vi "E2 Data Logger.vi"(7 "refnum in":refnum<file>) -> (3 "refnum out":refnum<file>)   [LabVIEW 2015]
uses:
  <vilib>/Rock Robotics/WPI/DriverStation/WPI_DriverStationRobotMode2.ctl
  Team Code/Robot Global Data.vi
  Moose Code/Auto_Conf.vi
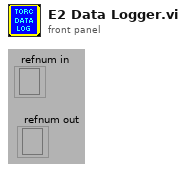
[diagram p1: front panel]
types:
  T1 = typedef "WPI_DriverStationRobotMode2.ctl" = enum16{"Autonomous Disabled", "Autonomous Enabled", "Teleop Disabled", "Teleop Enabled", "Disconnected", "Finish", "Test Disabled", "Test Enabled", "Emergency Stopped"}
  T2 = cluster{"LinearAcceleration X":dbl, "LinearAcceleration Y":dbl, "LinearAcceleration Z":dbl}
  T3 = cluster{"Velocity X":dbl, "Velocity Y":dbl, "Velocity Z":dbl, "Displacement X":dbl, "Displacement Y":dbl, "Displacement Z":dbl}
  T4 = enum16{"ResetBack", "ResetForward", "Reset", "Hold", "HighGoal", "LowGoal", "BumperShot", "EmergencyManualControl"}
  T5 = enum16{"ResetBack", "EmergencyManualControl", "ResetForward", "Hold", "Reset", "ManualControl"}
  T6 = cluster{"Yaw":dbl, "Roll":dbl, "Pitch":dbl, "Heading":dbl, "Fused Heading":dbl}
  T7 = typedef "WPI_SolenoidValue.ctl" = enum16{"Off", "On", "Forward", "Reverse"}
  T8 = typedef "WPI_CANTalonSRX_APIControlMode.ctl" = enum8{"Percent VBus", "Speed", "Position", "Slave", "Unchanged / Invalid", "Voltage Compensation", "Current", "Motion Profile"}
  T9 = enum16{"Empty", "Suck", "Hold", "LowGoal", "HighGoal", "BumperShot", "Shoot", "Dwell"}
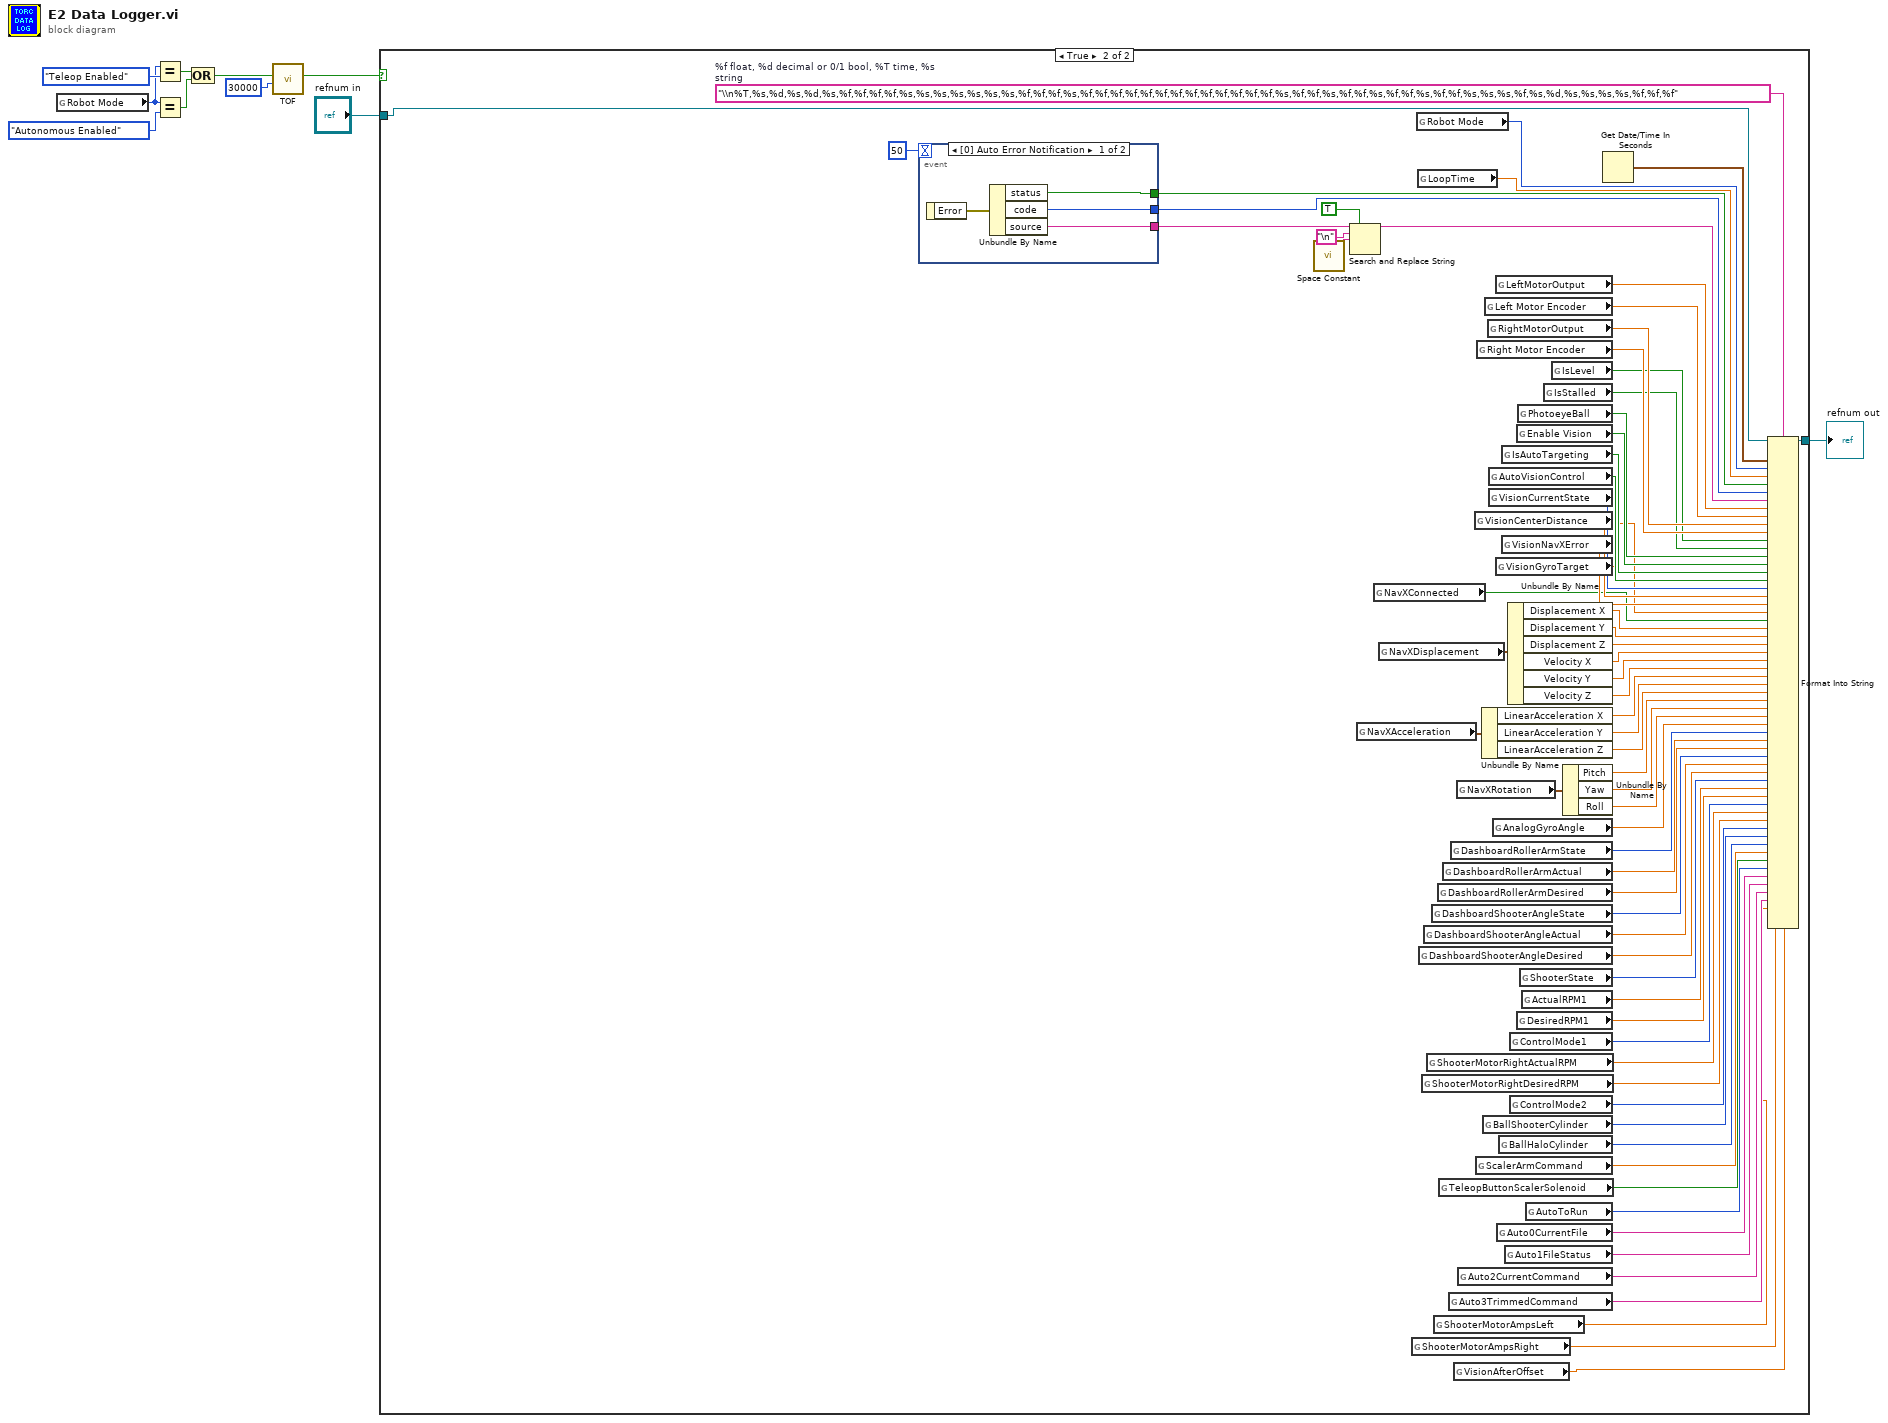
[diagram p0: block diagram]
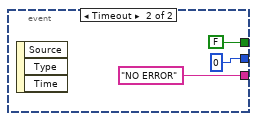
[diagram p3: hidden frame]
diagram:
  n1 = global read "Robot Global Data.vi" "Robot Mode"() -> (w4:T1)
  n2 = Equal?(x=w4, y=WPI_DriverStationRobotMode2."Teleop Enabled") -> (x = y?=w6:bool)
  n3 = Equal?(x=w4, y=WPI_DriverStationRobotMode2."Autonomous Enabled") -> (x = y?=w5:bool)
  n4 = Compound Arithmetic op=OR(w6, w5) -> (w3:bool)
  n5 = call "TOF.vi"("Delay (ms)"=u32 30000, "Input"=w3) -> ("Output"=w2:bool)  [unwired: 9 in]
  n6 = case shown="True" w2 {
    tunnel: [w11 w81] -> w10
    tunnel: "refnum in" -> [w11 w78]
    frame False {
    }
    frame True {
      w79 = "\\n%T,%s,%d,%s,%d,%s,%f,%f,%f,%f,%s,%s,%s,%s,%s,%s,%s,%f,%f,%f,%s,%f,%f,%f,%f,%f,%f,%f,%f,%f,%f,%f,%f,%f,%s,%f,%f,%s,%f,%f,%s,%f,%f,%s,%f,%f,%s,%s,%s,%f,%s,%d,%s,%s,%s,%s,%f,%f,%f"  # %f float, %d decimal or 0/1 bool, %T time, %s string
      n7 = event shown="[0] Auto Error Notification" {
        selector: _ -> [_ _]
        dyn-events: _ -> [_ _]
        timeout: 50 -> [_ _]
        tunnel: [w84 "NO ERROR" ("source")] -> w71
        tunnel: [w83 0 ("code")] -> w75
        tunnel: [w82 FALSE ("status")] -> w76
        event Auto Error Notification {
          n8 = event-data() -> ("Error"=w85:errorcluster)  [unwired: 1 in]
          n9 = Unbundle By Name(w85) -> ("status"=w82:bool, "code"=w83:i32, "source"=w84:string)
        }
        event Timeout {
          n10 = event-data() -> ()  [unwired: 1 in, 3 out]
        }
      }
      n11 = call <vilib>:"Space Constant.vi"() -> ("String"=w69:string)
      n12 = Search and Replace String(replace all?=TRUE ("replace all? (F)"), input string=w71, search string="\n", replace string=w69) -> (result string=w72:string)  [unwired: 4 in, 3 out]
      n13 = global read "Robot Global Data.vi" "NavXAcceleration"() -> (w73:T2)
      n14 = global read "Robot Global Data.vi" "NavXConnected"() -> (w52:bool)
      n15 = global read "Robot Global Data.vi" "NavXDisplacement"() -> (w51:T3)
      n16 = global read "Robot Global Data.vi" "ShooterMotorAmpsRight"() -> (w16:dbl)
      n17 = global read "Robot Global Data.vi" "Robot Mode"() -> (w18:T1)
      n18 = global read "Robot Global Data.vi" "LoopTime"() -> (w67:dbl)
      n19 = global read "Robot Global Data.vi" "DashboardShooterAngleDesired"() -> (w35:dbl)
      n20 = global read "Robot Global Data.vi" "ShooterMotorRightDesiredRPM"() -> (w29:dbl)
      n21 = global read "Robot Global Data.vi" "DashboardShooterAngleActual"() -> (w36:dbl)
      n22 = global read "Robot Global Data.vi" "ShooterMotorRightActualRPM"() -> (w30:dbl)
      n23 = global read "Robot Global Data.vi" "DashboardShooterAngleState"() -> (w37:T4)
      n24 = global read "Robot Global Data.vi" "ShooterMotorAmpsLeft"() -> (w17:dbl)
      n25 = global read "Robot Global Data.vi" "DashboardRollerArmDesired"() -> (w38:dbl)
      n26 = global read "Robot Global Data.vi" "TeleopButtonScalerSolenoid"() -> (w19:bool)
      n27 = global read "Robot Global Data.vi" "DashboardRollerArmActual"() -> (w39:dbl)
      n28 = global read "Auto_Conf.vi" "Auto3TrimmedCommand"() -> (w20:string)
      n29 = global read "Robot Global Data.vi" "DashboardRollerArmState"() -> (w40:T5)
      n30 = global read "Robot Global Data.vi" "VisionAfterOffset"() -> (w12:dbl)
      n31 = global read "Robot Global Data.vi" "NavXRotation"() -> (w74:T6)
      n32 = global read "Auto_Conf.vi" "Auto2CurrentCommand"() -> (w21:string)
      n33 = global read "Robot Global Data.vi" "VisionCenterDistance"() -> (w55:dbl)
      n34 = global read "Robot Global Data.vi" "ScalerArmCommand"() -> (w25:dbl)
      n35 = global read "Robot Global Data.vi" "Right Motor Encoder"() -> (w63:dbl)
      n36 = Unbundle By Name(w73) -> ("LinearAcceleration X"=w44:dbl, "LinearAcceleration Y"=w43:dbl, "LinearAcceleration Z"=w42:dbl)
      n37 = global read "Robot Global Data.vi" "BallShooterCylinder"() -> (w27:T7)
      n38 = global read "Robot Global Data.vi" "Left Motor Encoder"() -> (w65:dbl)
      n39 = global read "Robot Global Data.vi" "RightMotorOutput"() -> (w64:dbl)
      n40 = global read "Robot Global Data.vi" "AutoVisionControl"() -> (w57:bool)
      n41 = global read "Robot Global Data.vi" "VisionCurrentState"() -> (w56:enum16{"Disabled", "Enable", "Suspended", "PID"})
      n42 = global read "Robot Global Data.vi" "AnalogGyroAngle"() -> (w41:dbl)
      n43 = global read "Robot Global Data.vi" "LeftMotorOutput"() -> (w66:dbl)
      n44 = global read "Robot Global Data.vi" "VisionGyroTarget"() -> (w53:dbl)
      n45 = global read "Auto_Conf.vi" "Auto0CurrentFile"() -> (w23:string)
      n46 = global read "Robot Global Data.vi" "BallHaloCylinder"() -> (w26:T7)
      n47 = global read "Robot Global Data.vi" "IsAutoTargeting"() -> (w58:bool)
      n48 = global read "Robot Global Data.vi" "VisionNavXError"() -> (w54:dbl)
      n49 = global read "Auto_Conf.vi" "Auto1FileStatus"() -> (w22:string)
      n50 = Unbundle By Name(w51) -> ("Displacement X"=w50:dbl, "Displacement Y"=w49:dbl, "Displacement Z"=w48:dbl, "Velocity X"=w47:dbl, "Velocity Y"=w46:dbl, "Velocity Z"=w45:dbl)
      n51 = global read "Robot Global Data.vi" "ControlMode1"() -> (w31:T8)
      n52 = global read "Robot Global Data.vi" "ControlMode2"() -> (w28:T8)
      n53 = global read "Robot Global Data.vi" "Enable Vision"() -> (w59:bool)
      n54 = global read "Robot Global Data.vi" "DesiredRPM1"() -> (w32:dbl)
      n55 = global read "Robot Global Data.vi" "PhotoeyeBall"() -> (w60:bool)
      n56 = global read "Robot Global Data.vi" "ShooterState"() -> (w34:T9)
      n57 = global read "Robot Global Data.vi" "ActualRPM1"() -> (w33:dbl)
      n58 = global read "Auto_Conf.vi" "AutoToRun"() -> (w24:u8)
      n59 = global read "Robot Global Data.vi" "IsStalled"() -> (w61:bool)
      n60 = global read "Robot Global Data.vi" "IsLevel"() -> (w62:bool)
      n61 = Unbundle By Name(w74) -> ("Pitch"=w15:dbl, "Yaw"=w14:dbl, "Roll"=w13:dbl)
      n62 = Get Date/Time In Seconds() -> (seconds since 1Jan1904=w80:timestamp)
      n63 = Format Into String(format string=w79, initial string=w78, w80, w18, w67, w76, w75, w72, w66, w65, w64, w63, w62, w61, w60, w59, w58, w57, w56, w55, w54, w53, w52, w50, w49, w48, w47, w46, w45, w44, w43, w42, w15, w14, w13, w41, w40, w39, w38, w37, w36, w35, w34, w33, w32, w31, w30, w29, w28, w27, w26, w25, w19, w24, w23, w22, w21, w20, w17, w16, w12) -> (resulting string=w81:refnum<file>)  [unwired: 1 in, 1 out]
    }
  }
  "refnum out" <- w10
